vi "Navigation_Main_r1.2(new math for dist calc).vi"() -> ()   [LabVIEW 2015]
uses:
  <vilib>/myRIO/Common/Instrument Driver Framework/Utilities/typedefs/Generic FPGA Reference.ctl
  <vilib>/myRIO/Common/Instrument Driver Framework/Utilities/typedefs/myRIO v1.0 Reference.ctl
  <vilib>/myRIO/Common/Instrument Driver Framework/Utilities/typedefs/Hardware Version Enum.ctl
  <vilib>/myRIO/Common/Instrument Driver Framework/Utilities/typedefs/myRIO Generic Hardware Reference.ctl
  <vilib>/userdefined/High Color/nirio_resource_hc.ctl
  <vilib>/myRIO/Instrument Drivers/Onboard IO/PWM/typedefs/PWM Configuration.ctl
  <vilib>/myRIO/Instrument Drivers/Onboard IO/PWM/PWM.lvlib
  <vilib>/myRIO/Common/Instrument Driver Framework/myRIO v1.0/PWM/typedefs/PWM Channels Enum.ctl
  <vilib>/myRIO/Instrument Drivers/Onboard IO/PWM/typedefs/PWM Reference.ctl
  <vilib>/myRIO/Instrument Drivers/Onboard IO/PWM/vis/myRIO PWM Open.xnode
  <vilib>/myRIO/Common/Instrument Driver Framework/myRIO v1.0/PWM/vis/myRIO v1.1 Open PWM.vi
  <vilib>/rvi/interface/nirviOpenFPGA/nirviOpenFPGA.xnode
  <vilib>/myRIO/Instrument Drivers/Utilities/Utilities.lvlib
  <vilib>/rvi/interface/nirviReadWriteControl/nirviReadWriteControl.xnode
  NiFpgaLv.dll
  <vilib>/Utility/error.llb/Error Cluster From Error Code.vi
  <vilib>/rvi/interface/Simulation/niFpgaSimulationCallBeginRW.vi
  <vilib>/rvi/errors/niLvFpgaAdjustHostInterfaceError.vi
  Navi/E/FPGA Bitfiles/NavigationProjec_FPGATarget2_FPGAMainNavigati_PWPHW8gwDxI.lvbitx
  <vilib>/FPGAPlugInAG/myRIO-1900/niLvFpga_Open_myRIO-1900.vi
  <vilib>/rvi/interface/common/dynamic/niFpgaDynamicAddResources.vi
panel:
  out "max v":dbl
  out "v left wheel":dbl
  out "v right wheel":dbl
  out "Phi desired":dbl
  out "Omega":dbl format="%.2f"
  in  "Goal Position Y":dbl=5.0
  out "x position":dbl
  out "y position":dbl
  out "Scale":dbl=1.0
  out "Reset X Y":dbl
  out "Desired Velocity":dbl
  out "track width(ft)":dbl=4.0
  out "phi current":dbl
  out "robot desired velocity x component\n u1 (ft/s)":dbl
  out "robot desired velocity y component\n u2 (ft/s)":dbl
  out "RM Distance (ft)":dbl
  out "RR Distance (ft)":dbl
  out "LF Distance (ft)":dbl
  out "LM Distance (ft)":dbl
  out "RF Distance (ft)":dbl
  out "LR Distance (ft)":dbl
  out "Tick Count(mSec) 2":u32 caption="Tick Count(mSec)"
  out "Right Setpoint":dbl
  out "Left Setpoint":dbl
  in  "Start Position Y":dbl=5.0
  in  "Goal Position X":dbl=5.0
  in  "Start Position X":dbl=1.0
  in  "All Stop":bool
  in  "Left Side PID Gains":T1={"proportional gain (Kc)"=0.002, "integral time (Ti, min)"=7e-07, "derivative time (Td, min)"=0.0} {"derivative time (Td, min)" format="%.8f"; "integral time (Ti, min)" format="%.8f"; "proportional gain (Kc)" format="%.8f"}
  in  "Left Side Output Range":cluster{"output high":dbl, "output low":dbl}={"output high"=0.13333, "output low"=-0.13333} {"output low" format="%.5f"; "output high" format="%.5f"}
  in  "Right Side PID Gains":T1={"proportional gain (Kc)"=0.002, "integral time (Ti, min)"=7e-07, "derivative time (Td, min)"=0.0} {"derivative time (Td, min)" format="%.8f"; "integral time (Ti, min)" format="%.8f"; "proportional gain (Kc)" format="%.8f"}
  in  "Right Side Output Range":cluster{"output high":dbl, "output low":dbl}={"output high"=0.13333, "output low"=-0.13333} {"output low" format="%.5f"; "output high" format="%.5f"}
  out "Left PWM":dbl
  out "Right PWM":dbl
  out "LF Rot Velocity (rot/s)":dbl
  out "LM Rot Velocity (rot/s)":dbl
  out "LR Rot Velocity (rot/s)":dbl
  out "RR Rot Velocity (rot/s)":dbl
  out "RM Linear Velocity (rot/s)":dbl
  out "RF Linear Velocity (rot/s)":dbl
  in  "Encoder Reset":bool
  out "SYS.SELECTA":u8 format="%08b"
  out "ENC.B_c.CNTR":i32
  out "ENC.B_b.CNTR":i32
  out "ENC.B_a.CNTR":i32
  out "ENC.A_c.CNTR":i32
  out "ENC.A_b.CNTR":i32
  out "ENC.A_a.CNTR":i32
  out "Current Rot Velocity (rot/s)":T2(graph)
  # "Motor Control Parameters"
  # "Press Go when Start and Goal Are Set"
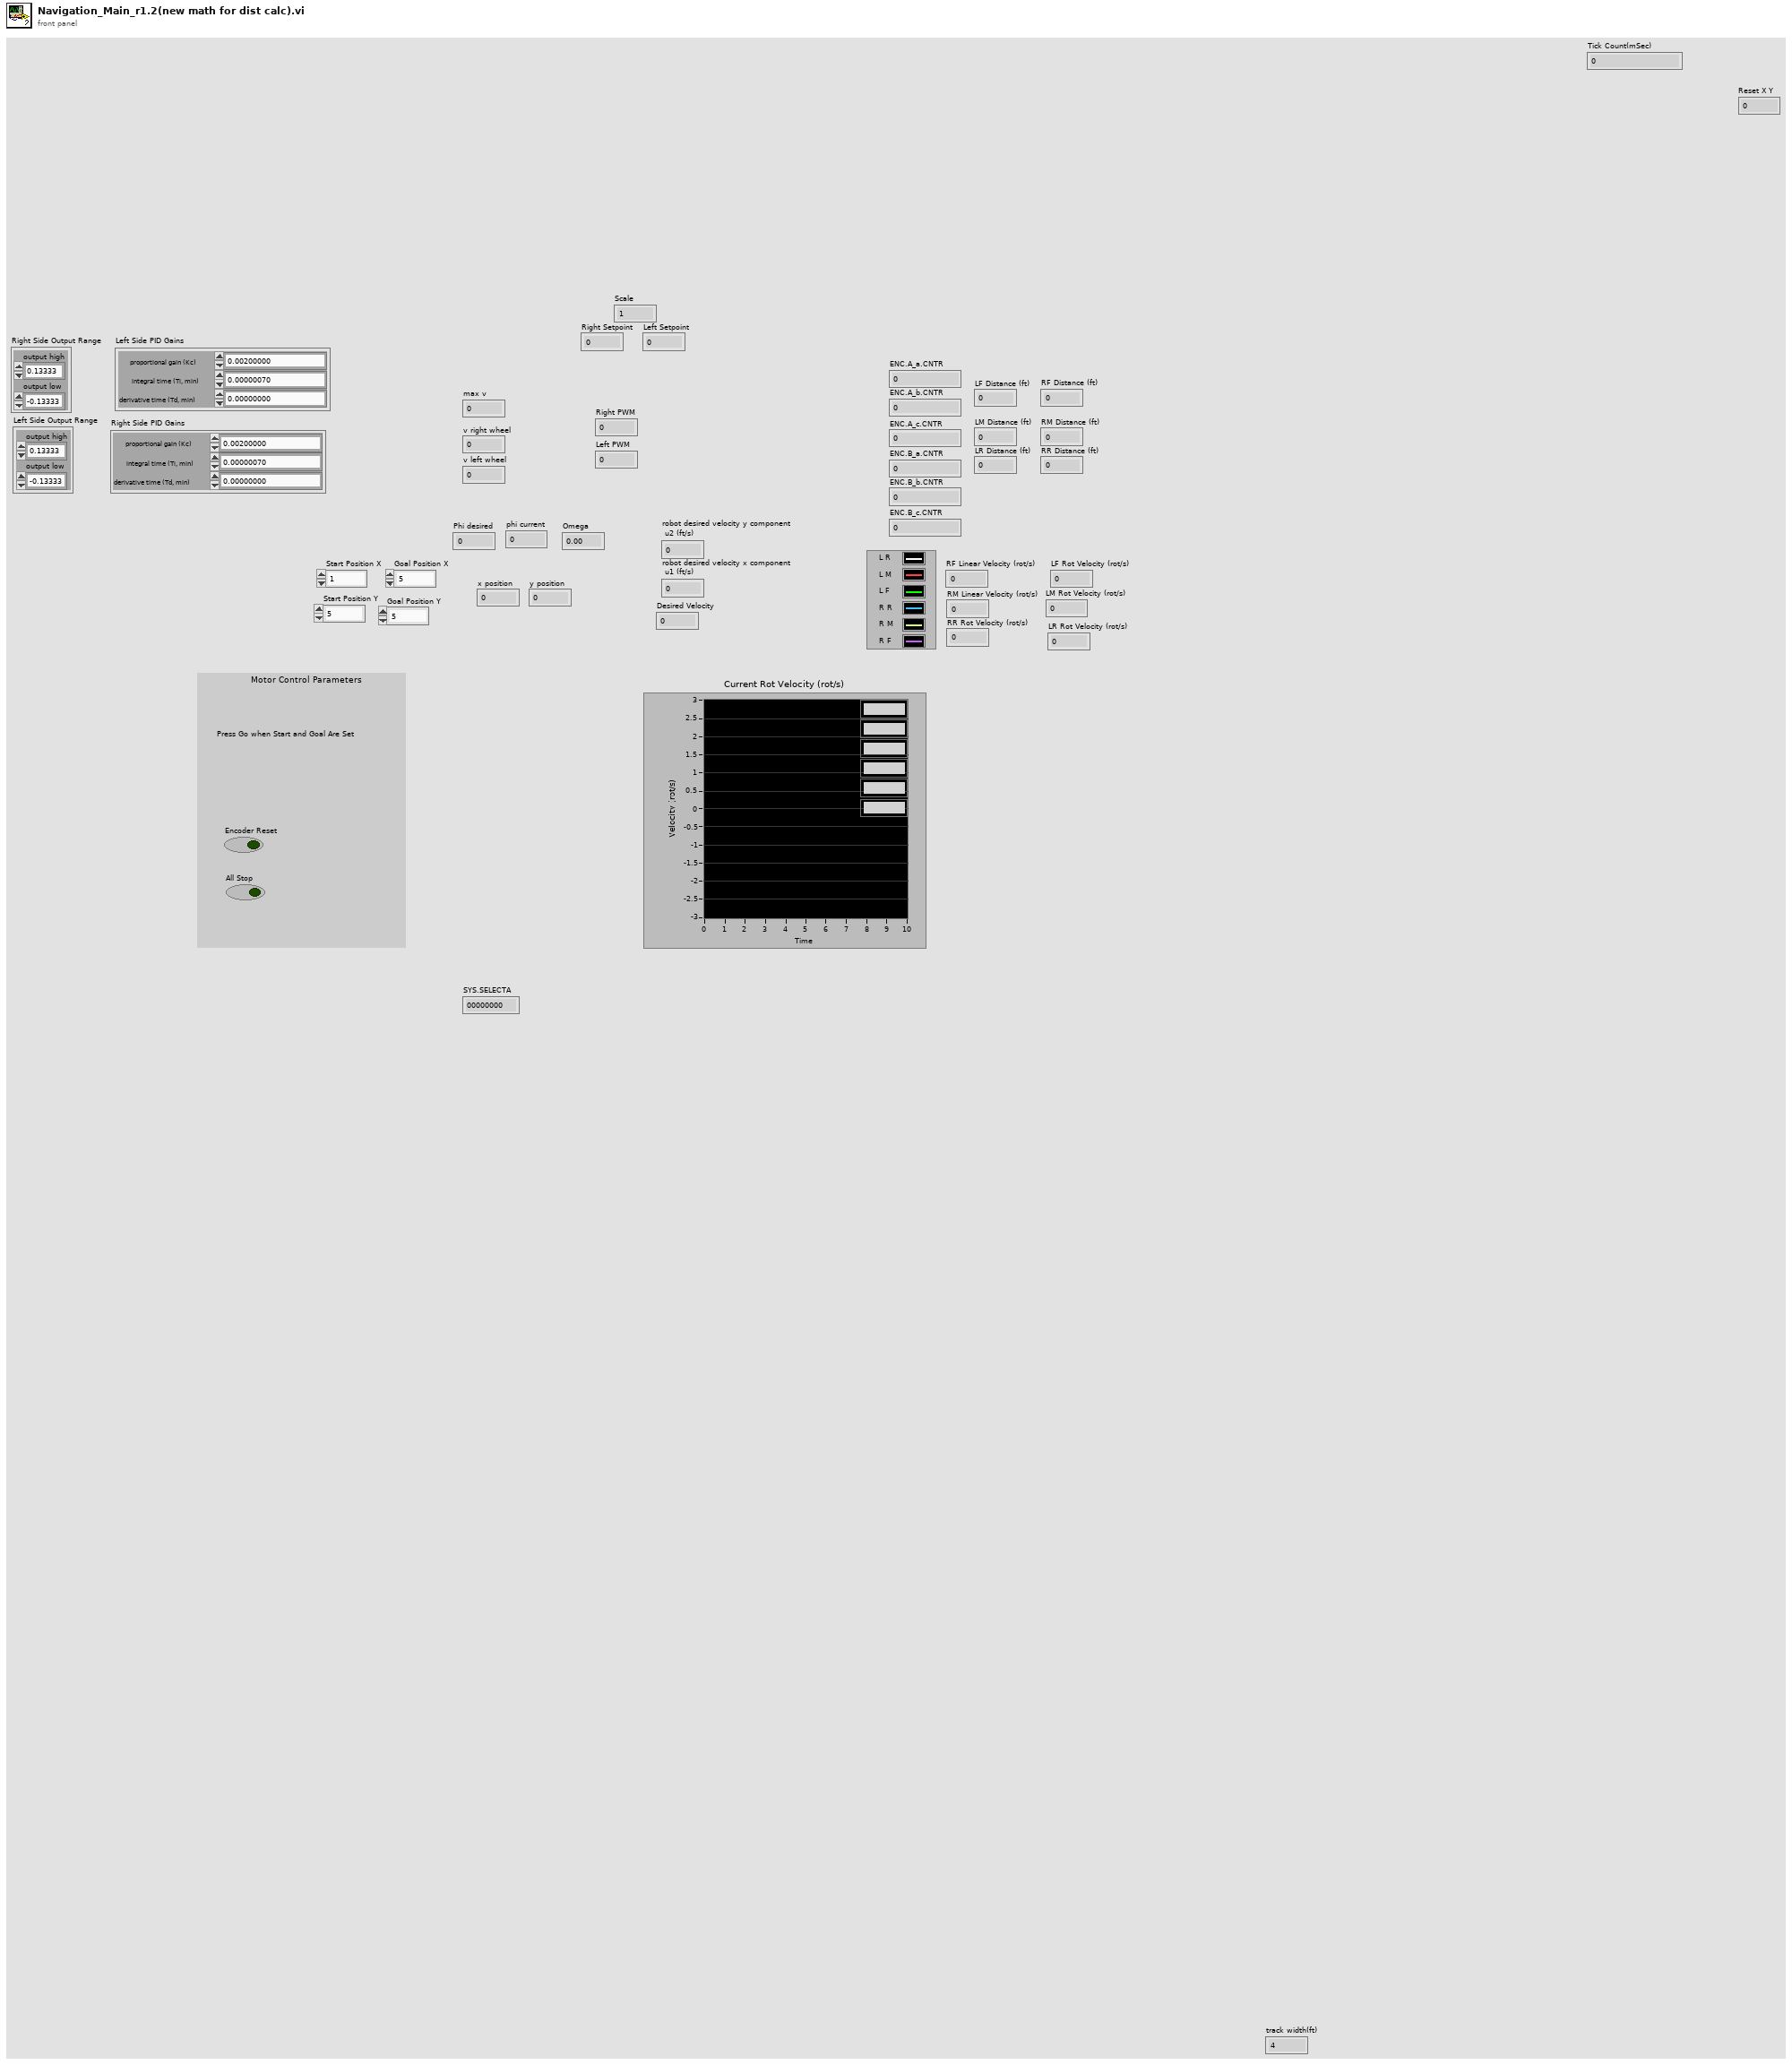
[diagram p1: front panel]
types:
  T1 = cluster{"proportional gain (Kc)":dbl, "integral time (Ti, min)":dbl, "derivative time (Td, min)":dbl}
  T2 = cluster{"Rotational Velocity (RPS)":dbl, "Rotational Velocity (RPS)":dbl, "Rotational Velocity (RPS)":dbl, "Rotational Velocity (RPS)":dbl, "Rotational Velocity (RPS)":dbl, "Rotational Velocity (RPS)":dbl}
  T3 = typedef "nirio_resource_hc.ctl" = tag
  T4 = typedef "Hardware Version Enum.ctl" = enum16{"Unknown", "myRIO-1900", "myRIO-1950", "roboRIO"}
  T5 = typedef "PWM.lvlib/PWM Reference.ctl" = cluster{"myRIO Reference":T6, "PWM Channels Enum":T9, "PWM Configuration":T10}
  T6 = typedef "myRIO Generic Hardware Reference.ctl" = cluster{"myRIO Model":T4, "myRIO Hardware Reference":T7}
  T7 = typedef "myRIO v1.0 Reference.ctl" = cluster{"Generic FPGA Reference":T8, "Allow multiple opens":bool}
  T8 = typedef "Generic FPGA Reference.ctl" = refnum<k20>
  T9 = typedef "PWM Channels Enum.ctl" = enum16{"Not Connected", "C/PWM0", "C/PWM1", "A/PWM0", "A/PWM1", "A/PWM2", "B/PWM0", "B/PWM1", "B/PWM2", "PWM/PWM0", "PWM/PWM1", "PWM/PWM2", "PWM/PWM3", "PWM/PWM4", "PWM/PWM5", "PWM/PWM6", "PWM/PWM7", "PWM/PWM8", "PWM/PWM9"}
  T10 = typedef "PWM.lvlib/PWM Configuration.ctl" = cluster{"Frequency":dbl, "Duty Cycle":dbl}
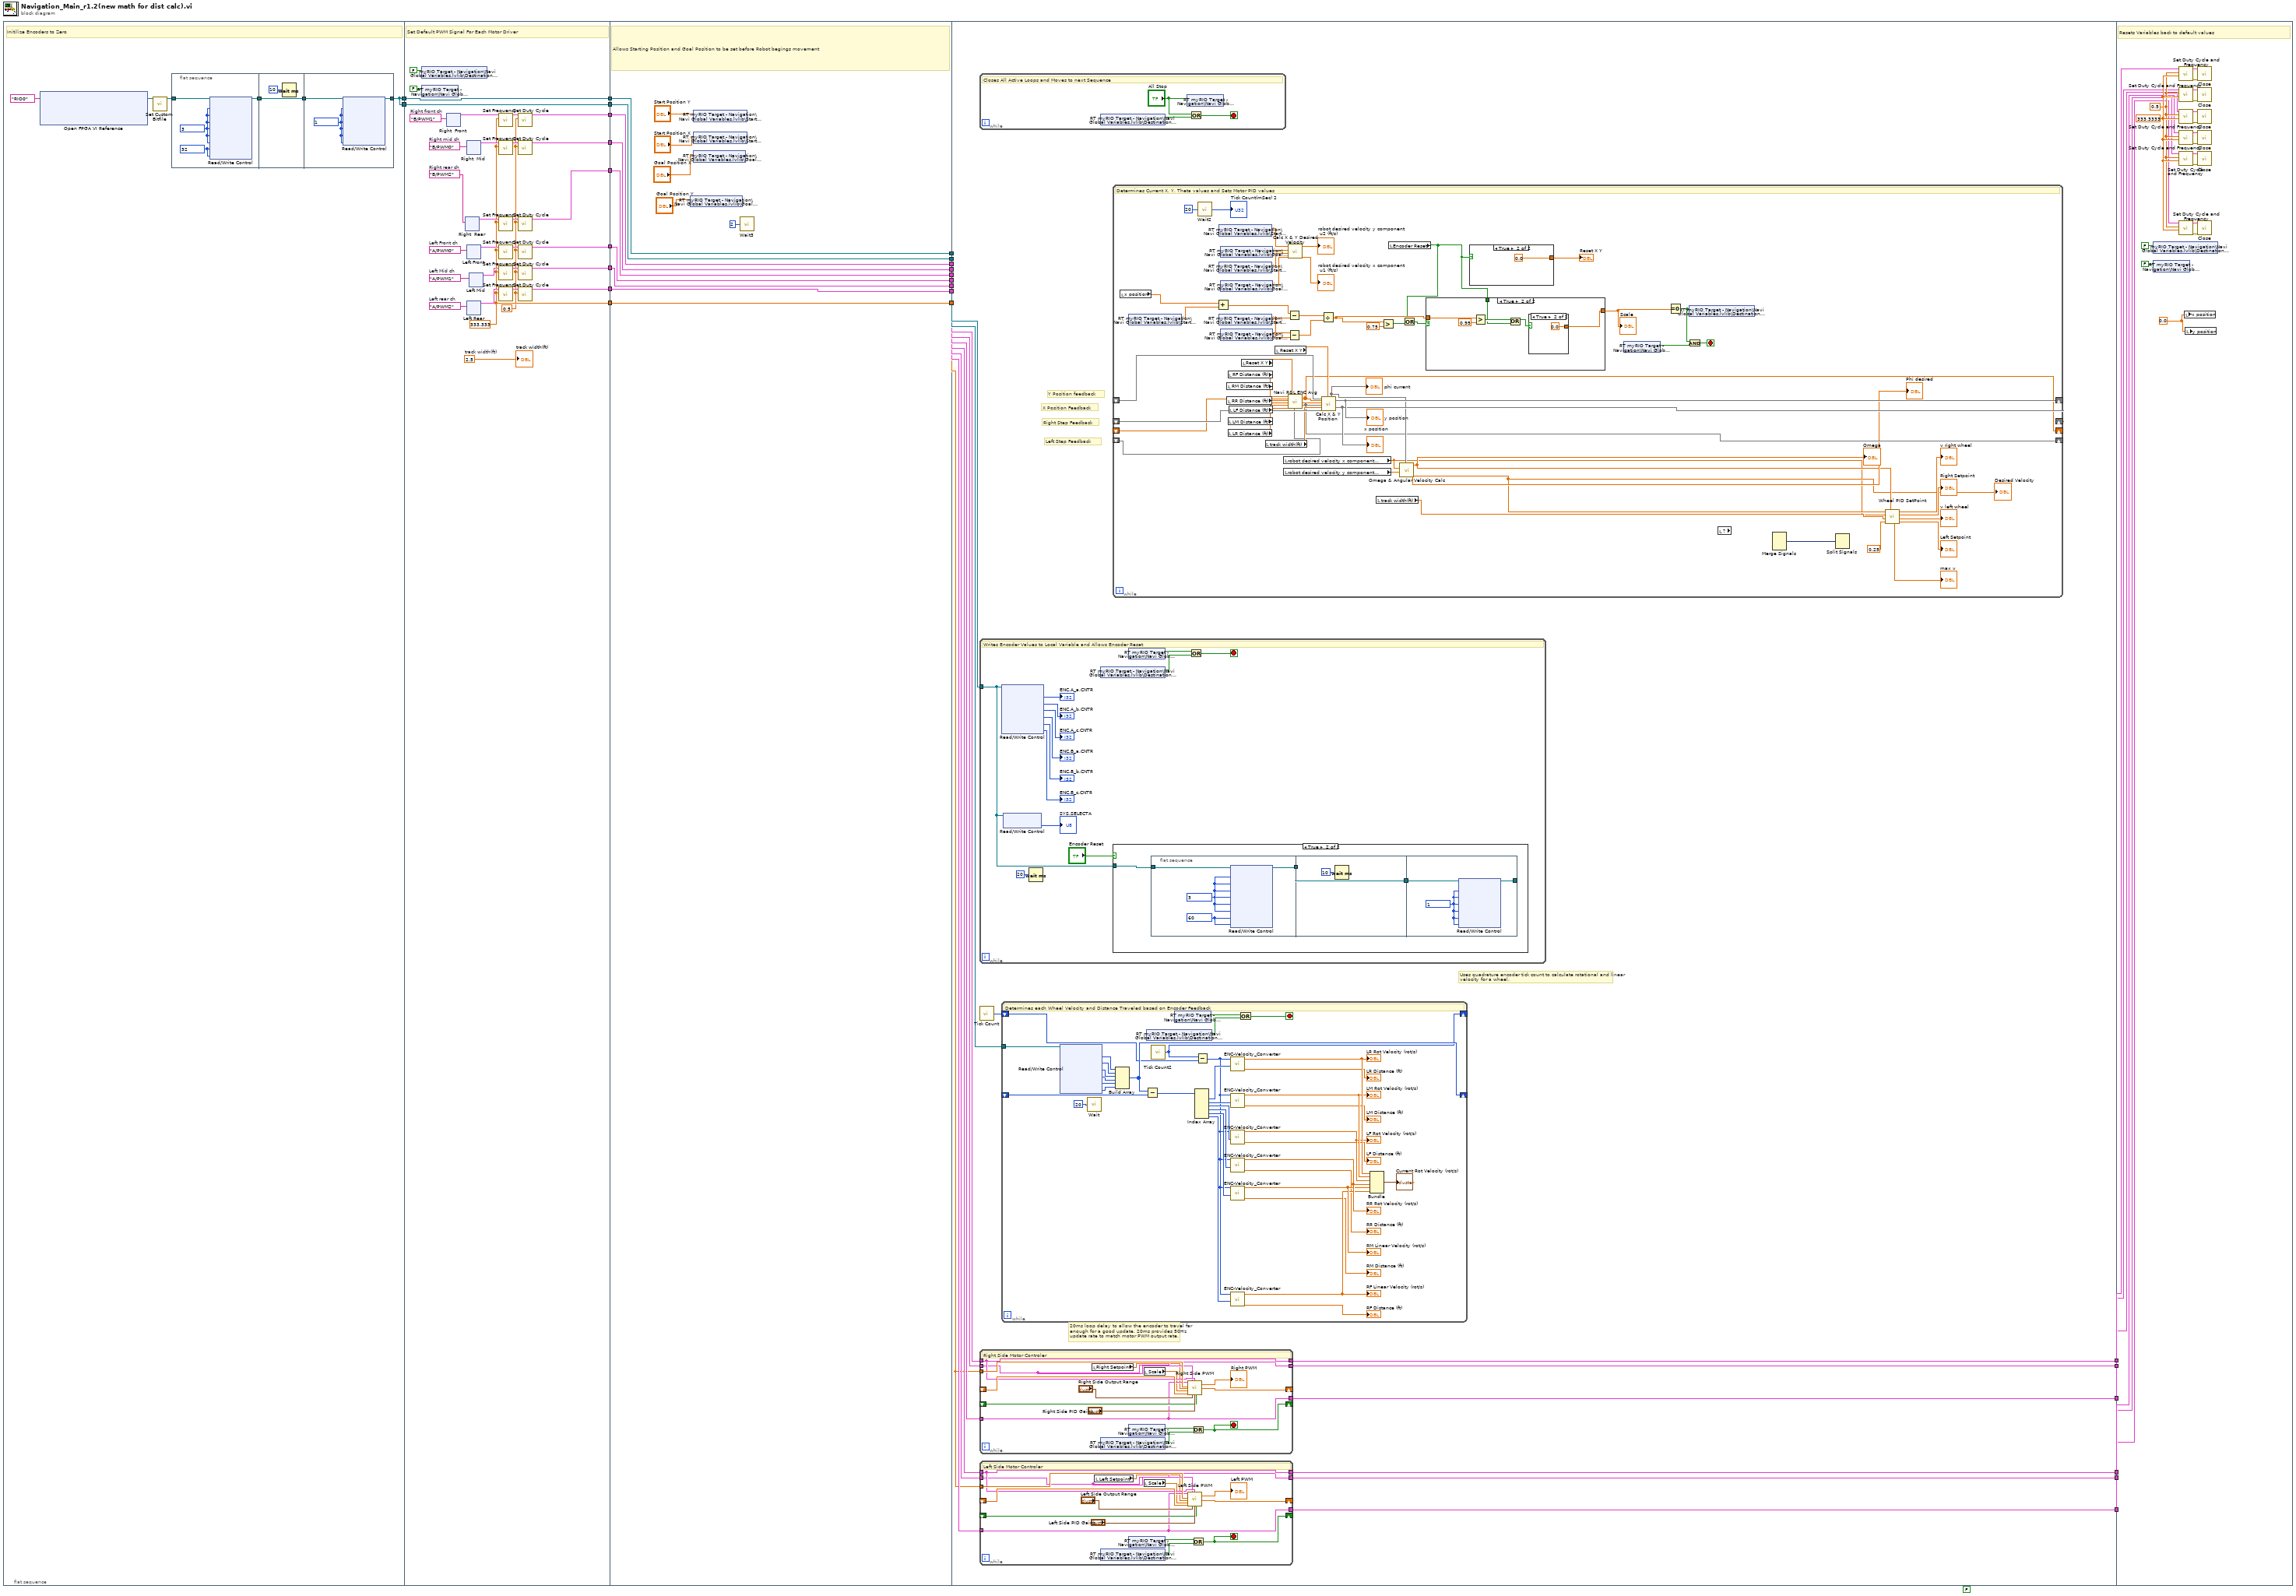
[diagram p0: block diagram]
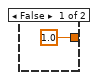
[diagram p2: hidden frame]
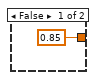
[diagram p3: hidden frame]
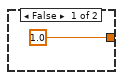
[diagram p4: hidden frame]
diagram:
  (unwired) FALSE ("stop")
  n1 = flat-sequence {
    tunnel: [w29] -> w26
    tunnel: [w29] -> w25
    tunnel: [w60] -> w24
    tunnel: [w55] -> w23
    tunnel: [w51] -> w22
    tunnel: [w50] -> w21
    tunnel: [w49] -> w20
    tunnel: [w48] -> w19
    tunnel: [w47] -> w18
    tunnel: [w46] -> w17
    tunnel: w26 -> [w45]
    tunnel: [w45] -> w16
    tunnel: w25 -> [w46]
    tunnel: w24 -> [w182]
    tunnel: [w182] -> w15
    tunnel: w23 -> [w181]
    tunnel: [w181] -> w14
    tunnel: w22 -> [w180]
    tunnel: [w180] -> w13
    tunnel: w21 -> [w179]
    tunnel: [w179] -> w12
    tunnel: w20 -> [w178]
    tunnel: [w178] -> w11
    tunnel: w19 -> [w177]
    tunnel: [w177] -> w10
    tunnel: w18 -> [w176]
    tunnel: [w176] -> w9
    tunnel: w17 -> [w175]
    tunnel: [w175] -> w8
    tunnel: w16 -> [w174]
    tunnel: [w174] -> w7
    tunnel: w15 -> [w189]
    tunnel: w14 -> [w190]
    tunnel: w13 -> [w195]
    tunnel: w12 -> [w194]
    tunnel: w11 -> [w193]
    tunnel: w10 -> [w192]
    tunnel: w9 -> [w191]
    tunnel: w8 -> [w197]
    tunnel: w7 -> [w196]
    tunnel: [w188] -> w6
    tunnel: [w187] -> w5
    tunnel: [w186] -> w4
    tunnel: [w185] -> w3
    tunnel: [w184] -> w2
    tunnel: [w183] -> w1
    tunnel: w6 -> [w369]
    tunnel: w5 -> [w368]
    tunnel: w4 -> [w367]
    tunnel: w3 -> [w366]
    tunnel: w2 -> [w365]
    tunnel: w1 -> [w364]
    frame #0 {
      # "Initilize Encoders to Zero"
      n2 = xnode "Open FPGA VI Reference"("resource name"=tag "RIO0") -> ("FPGA VI Reference Out"=w28:refnum<k20>)  [unwired: 1 in, 1 out]
      n3 = call <vilib>:"Set Custom Bitfile.vi"("Custom FPGA Reference In"=w28) -> ("Custom FPGA Reference Out"=w30:refnum<k20>)  [unwired: 9 in, 1 out]
      n4 = flat-sequence {
        tunnel: w30 -> [w35]
        tunnel: [w33] -> w32
        tunnel: w32 -> [w37]
        tunnel: [w37] -> w31
        tunnel: w31 -> [w40]
        tunnel: [w39] -> w29
        frame #0 {
          w34 = u8 32 ("SYS.SELECTA")
          w36 = u8 3 ("ENC.B_c.CNFG")
          n5 = xnode "Read/Write Control"("FPGA VI Reference In"=w35, "ENC.A_a.CNFG"=w36, "ENC.A_b.CNFG"=w36, "ENC.A_c.CNFG"=w36, "ENC.B_a.CNFG"=w36, "ENC.B_b.CNFG"=w36, "ENC.B_c.CNFG"=w36, "SYS.SELECTA"=w34, "SYS.SELECTB"=w34) -> ("FPGA VI Reference Out"=w33:refnum<k20>)  [unwired: 1 in, 1 out]
        }
        frame #1 {
          n6 = Wait (ms)(milliseconds to wait=u32 10) -> ()  [unwired: 1 out]
        }
        frame #2 {
          w41 = u8 1 ("ENC.B_c.CNFG")
          n7 = xnode "Read/Write Control"("FPGA VI Reference In"=w40, "ENC.A_a.CNFG"=w41, "ENC.A_b.CNFG"=w41, "ENC.A_c.CNFG"=w41, "ENC.B_a.CNFG"=w41, "ENC.B_b.CNFG"=w41, "ENC.B_c.CNFG"=w41) -> ("FPGA VI Reference Out"=w39:refnum<k20>)  [unwired: 1 in, 1 out]
        }
      }
    }
    frame #1 {
      w42 = 2.5  # track width(ft)
      w52 = 0.5 ("Duty Cycle")
      w60 = 333.333 ("Frequency [Hz]")
      w67 = tag "B/PWM2"  # Right rear ch
      w68 = tag "B/PWM0"  # Right mid ch
      w69 = tag "B/PWM1"  # Right front ch
      w70 = tag "A/PWM2"  # Left rear ch
      w71 = tag "A/PWM0"  # Left Front ch
      w72 = tag "A/PWM1"  # Left Mid ch
      # "Set Default PWM Signal For Each Motor Driver"
      n8 = shared-variable "RT myRIO Target - Navigation\\Navi Global Variables.lvlib\\Destination Reached"(FALSE) -> ()  [unwired: 1 in, 1 out]
      n9 = shared-variable "RT myRIO Target - Navigation\\Navi Global Variables.lvlib\\All Stop"(FALSE) -> ()  [unwired: 1 in, 1 out]
      n10 = xnode "Right  Front"("Channel Name"=w69) -> ("PWM Ref Out"=w63:T5)  [unwired: 2 in, 1 out]
      n11 = xnode "Right  Rear"("Channel Name"=w67) -> ("PWM Ref Out"=w61:T5)  [unwired: 2 in, 1 out]
      n12 = xnode "Right  Mid"("Channel Name"=w68) -> ("PWM Ref Out"=w62:T5)  [unwired: 2 in, 1 out]
      n13 = xnode "Left Front"("Channel Name"=w71) -> ("PWM Ref Out"=w65:T5)  [unwired: 2 in, 1 out]
      n14 = xnode "Left Rear"("Channel Name"=w70) -> ("PWM Ref Out"=w64:T5)  [unwired: 2 in, 1 out]
      n15 = xnode "Left Mid"("Channel Name"=w72) -> ("PWM Ref Out"=w66:T5)  [unwired: 2 in, 1 out]
      n16 = call <vilib>:"Set Frequency.vi"("Frequency [Hz]"=w60, "PWM Ref In"=w63) -> ("PWM Ref Out"=w56:T5)  [unwired: 7 in, 1 out]
      n17 = call <vilib>:"Set Frequency.vi"("Frequency [Hz]"=w60, "PWM Ref In"=w62) -> ("PWM Ref Out"=w57:T5)  [unwired: 7 in, 1 out]
      n18 = call <vilib>:"Set Frequency.vi"("Frequency [Hz]"=w60, "PWM Ref In"=w61) -> ("PWM Ref Out"=w58:T5)  [unwired: 7 in, 1 out]
      n19 = call <vilib>:"Set Frequency.vi"("Frequency [Hz]"=w60, "PWM Ref In"=w65) -> ("PWM Ref Out"=w53:T5)  [unwired: 7 in, 1 out]
      n20 = call <vilib>:"Set Frequency.vi"("Frequency [Hz]"=w60, "PWM Ref In"=w66) -> ("PWM Ref Out"=w59:T5)  [unwired: 7 in, 1 out]
      n21 = call <vilib>:"Set Frequency.vi"("Frequency [Hz]"=w60, "PWM Ref In"=w64) -> ("PWM Ref Out"=w54:T5)  [unwired: 7 in, 1 out]
      n22 = call <vilib>:"Set Duty Cycle.vi"("Duty Cycle"=w52, "PWM Ref In"=w56) -> ("PWM Ref Out"=w51:T5)  [unwired: 7 in, 1 out]
      n23 = call <vilib>:"Set Duty Cycle.vi"("Duty Cycle"=w52, "PWM Ref In"=w57) -> ("PWM Ref Out"=w50:T5)  [unwired: 7 in, 1 out]
      n24 = call <vilib>:"Set Duty Cycle.vi"("Duty Cycle"=w52, "PWM Ref In"=w58) -> ("PWM Ref Out"=w49:T5)  [unwired: 7 in, 1 out]
      n25 = call <vilib>:"Set Duty Cycle.vi"("Duty Cycle"=w52, "PWM Ref In"=w53) -> ("PWM Ref Out"=w48:T5)  [unwired: 7 in, 1 out]
      n26 = call <vilib>:"Set Duty Cycle.vi"("Duty Cycle"=w52, "PWM Ref In"=w59) -> ("PWM Ref Out"=w47:T5)  [unwired: 7 in, 1 out]
      n27 = call <vilib>:"Set Duty Cycle.vi"("Duty Cycle"=w52, "PWM Ref In"=w54) -> ("PWM Ref Out"=w55:T5)  [unwired: 7 in, 1 out]
      "track width(ft)" <- w42
    }
    frame #2 {
      # "Allows Starting Position and Goal Position to be set before Robot begings movement"
      n28 = shared-variable "RT myRIO Target - Navigation\\Navi Global Variables.lvlib\\Goal Position Y"("Goal Position Y") -> ()  [unwired: 1 in, 1 out]
      n29 = shared-variable "RT myRIO Target - Navigation\\Navi Global Variables.lvlib\\Start Position Y"("Start Position Y") -> ()  [unwired: 1 in, 1 out]
      n30 = shared-variable "RT myRIO Target - Navigation\\Navi Global Variables.lvlib\\Start Position X"("Start Position X") -> ()  [unwired: 1 in, 1 out]
      n31 = shared-variable "RT myRIO Target - Navigation\\Navi Global Variables.lvlib\\Goal Position X"("Goal Position X") -> ()  [unwired: 1 in, 1 out]
      n32 = call "Wait3"("Count(mSec)"=u32 2) -> ()  [unwired: 1 out]
    }
    frame #3 {
      # "Left Step Feedback"
      # "Y Position feedback"
      # "Right Step Feedback"
      # "X Position Feedback"
      # "Uses quadrature encoder tick count to calculate rotational and linear velocity for a wheel."
      # "20ms loop delay to allow the encoder to travel far enough for a good update. 20ms provides 50Hz update rate to match motor PWM output rate."
      n33 = while {
        stop <- w269 stop-if-true
        # "Closes All Active Loops and Moves to next Sequence"
        n34 = shared-variable "RT myRIO Target - Navigation\\Navi Global Variables.lvlib\\Destination Reached"() -> (w267:bool)  [unwired: 1 in, 1 out]
        n35 = shared-variable "RT myRIO Target - Navigation\\Navi Global Variables.lvlib\\All Stop"("All Stop") -> ()  [unwired: 1 in, 1 out]
        n36 = Or(x="All Stop", y=w267) -> (x .or. y?=w269:bool)
      }
      n37 = while {
        tunnel: w197 -> [w303]
        stop <- w300 stop-if-true
        # "Writes Encoder Values to Local Variable and Allows Encoder Reset"
        n38 = xnode "Read/Write Control"("FPGA VI Reference In"=w303) -> ("ENC.A_a.CNTR"=→"ENC.A_a.CNTR":u32, "ENC.A_b.CNTR"=→"ENC.A_b.CNTR":u32, "ENC.A_c.CNTR"=→"ENC.A_c.CNTR":u32, "ENC.B_a.CNTR"=→"ENC.B_a.CNTR":u32, "ENC.B_b.CNTR"=→"ENC.B_b.CNTR":u32, "ENC.B_c.CNTR"=→"ENC.B_c.CNTR":u32)  [unwired: 1 in, 2 out]
        n39 = xnode "Read/Write Control"("FPGA VI Reference In"=w303) -> ("SYS.SELECTA"=→"SYS.SELECTA":u8)  [unwired: 1 in, 2 out]
        n40 = Wait (ms)(milliseconds to wait=u32 20) -> ()  [unwired: 1 out]
        n41 = shared-variable "RT myRIO Target - Navigation\\Navi Global Variables.lvlib\\Destination Reached"() -> (w302:bool)  [unwired: 1 in, 1 out]
        n42 = case shown="True" "Encoder Reset" {
          tunnel: w303 -> [_ w313]
          frame False {
          }
          frame True {
            n43 = flat-sequence {
              tunnel: w313 -> [w318]
              tunnel: [w316] -> w315
              tunnel: w315 -> [w320]
              tunnel: [w320] -> w314
              tunnel: w314 -> [w323]
              tunnel: [w322] -> _
              frame #0 {
                w317 = u8 60 ("SYS.SELECTA")
                w319 = u8 3 ("ENC.B_c.CNFG")
                n44 = xnode "Read/Write Control"("FPGA VI Reference In"=w318, "ENC.A_a.CNFG"=w319, "ENC.A_b.CNFG"=w319, "ENC.A_c.CNFG"=w319, "ENC.B_a.CNFG"=w319, "ENC.B_b.CNFG"=w319, "ENC.B_c.CNFG"=w319, "SYS.SELECTA"=w317, "SYS.SELECTB"=w317) -> ("FPGA VI Reference Out"=w316:refnum<k20>)  [unwired: 1 in, 1 out]
              }
              frame #1 {
                n45 = Wait (ms)(milliseconds to wait=u32 10) -> ()  [unwired: 1 out]
              }
              frame #2 {
                w324 = u8 1 ("ENC.B_c.CNFG")
                n46 = xnode "Read/Write Control"("FPGA VI Reference In"=w323, "ENC.A_a.CNFG"=w324, "ENC.A_b.CNFG"=w324, "ENC.A_c.CNFG"=w324, "ENC.B_a.CNFG"=w324, "ENC.B_b.CNFG"=w324, "ENC.B_c.CNFG"=w324) -> ("FPGA VI Reference Out"=w322:refnum<k20>)  [unwired: 1 in, 1 out]
              }
            }
          }
        }
        n47 = shared-variable "RT myRIO Target - Navigation\\Navi Global Variables.lvlib\\All Stop"() -> (w301:bool)  [unwired: 1 in, 1 out]
        n48 = Or(x=w301, y=w302) -> (x .or. y?=w300:bool)
      }
      n49 = call "Tick Count"() -> ("Tick Count(uSec)"=w198:u32)
      n50 = while {
        tunnel: w195 -> [w292]
        tunnel: w194 -> [w291]
        tunnel: w193 -> [w290]
        tunnel: w189 -> [w299]
        shift-right: [w295] -> _
        shift-left: _ -> [w294]
        shift-right: [w287] -> _
        shift-left: _ -> [w293]
        tunnel: [w292] -> w188
        tunnel: [w291] -> w187
        tunnel: [w290] -> w186
        stop <- w287 stop-if-true
        # "Right Side Motor Controler"
        n51 = local read "Right Setpoint"() -> (w286:dbl)
        n52 = shared-variable "RT myRIO Target - Navigation\\Navi Global Variables.lvlib\\Destination Reached"() -> (w289:bool)  [unwired: 1 in, 1 out]
        n53 = shared-variable "RT myRIO Target - Navigation\\Navi Global Variables.lvlib\\All Stop"() -> (w288:bool)  [unwired: 1 in, 1 out]
        n54 = local read "Scale"() -> (w285:dbl)
        n55 = call "Right Side PWM.vi"("Right rear"=w290, "Frequency"=w299, "Right Side Setpoint"=w286, "Right Side Scale"=w285, "Right PID Feedback"=w294, "Right Mid"=w291, "Right Side Output Range"="Right Side Output Range", "Right Front"=w292, "Right Side PID Gains"="Right Side PID Gains", "Reset Right E.T."=w293) -> ("Right PWM"=→"Right PWM":dbl, "Right PID Output"=w295:dbl)  [unwired: 8 in]
        n56 = Or(x=w288, y=w289) -> (x .or. y?=w287:bool)
      }
      n57 = while {
        tunnel: w192 -> [w277]
        tunnel: w191 -> [w276]
        tunnel: w190 -> [w275]
        tunnel: w189 -> [w284]
        shift-right: [w280] -> _
        shift-left: _ -> [w279]
        shift-right: [w272] -> _
        shift-left: _ -> [w278]
        tunnel: [w277] -> w185
        tunnel: [w276] -> w184
        tunnel: [w275] -> w183
        stop <- w272 stop-if-true
        # "Left Side Motor Controler"
        n58 = local read "Left Setpoint"() -> (w271:dbl)
        n59 = shared-variable "RT myRIO Target - Navigation\\Navi Global Variables.lvlib\\Destination Reached"() -> (w274:bool)  [unwired: 1 in, 1 out]
        n60 = shared-variable "RT myRIO Target - Navigation\\Navi Global Variables.lvlib\\All Stop"() -> (w273:bool)  [unwired: 1 in, 1 out]
        n61 = local read "Scale"() -> (w270:dbl)
        n62 = call "Left Side PWM.vi"("Left rear"=w275, "Frequency"=w284, "Left Side Setpoint"=w271, "Left Side Scale"=w270, "Left PID Feedback"=w279, "Left Mid"=w276, "Left Side Output Range"="Left Side Output Range", "Left Front"=w277, "Left Side PID Gains"="Left Side PID Gains", "Reset Left E.T."=w278) -> ("Left PWM"=→"Left PWM":dbl, "Left PID Output"=w280:dbl)  [unwired: 8 in]
        n63 = Or(x=w273, y=w274) -> (x .or. y?=w272:bool)
      }
      n64 = while {
        shift-right: [w352] -> _
        shift-left: _ -> [w351]
        shift-right: [w349] -> _
        shift-left: w198 -> [w348]
        tunnel: w196 -> [w359]
        stop <- w344 stop-if-true
        # "Determines each Wheel Velocity and Distance Traveled based on Encoder Feedback"
        n65 = xnode "Read/Write Control"("FPGA VI Reference In"=w359) -> ("ENC.A_a.CNTR"=w358:u32, "ENC.A_b.CNTR"=w357:u32, "ENC.A_c.CNTR"=w356:u32, "ENC.B_a.CNTR"=w355:u32, "ENC.B_b.CNTR"=w354:u32, "ENC.B_c.CNTR"=w353:u32)  [unwired: 1 in, 2 out]
        n66 = call "Wait"("Count(mSec)"=u32 20) -> ()  [unwired: 1 out]
        n67 = Build Array(w358, w357, w356, w355, w354, w353) -> (w352:u32[])
        n68 = Subtract(x=w352, y=w351) -> (x-y=w350:u32[])
        n69 = shared-variable "RT myRIO Target - Navigation\\Navi Global Variables.lvlib\\Destination Reached"() -> (w346:bool)  [unwired: 1 in, 1 out]
        n70 = call "Tick Count2"() -> ("Tick Count(uSec)"=w349:u32)
        n71 = shared-variable "RT myRIO Target - Navigation\\Navi Global Variables.lvlib\\All Stop"() -> (w345:bool)  [unwired: 1 in, 1 out]
        n72 = Index Array(array=w350) -> (element #1=w343:u32, element #2=w340:u32, element #3=w338:u32, element #4=w336:u32, element #5=w334:u32, element #6=w331:u32)  [unwired: 6 in]
        n73 = Subtract(x=w349, y=w348) -> (x-y=w332:u32)
        n74 = call "ENC-Velocity_Converter.vi"("delta  Encoder Count"=w343, "dt (uSec)"=w332) -> ("Distance (ft)"=→"LR Distance (ft)":dbl, "Rotational Velocity (RPS)"=w342:dbl)  [unwired: 7 in, 1 out]
        "LR Rot Velocity (rot/s)" <- w342
        n75 = call "ENC-Velocity_Converter.vi"("delta  Encoder Count"=w340, "dt (uSec)"=w332) -> ("Distance (ft)"=→"LM Distance (ft)":dbl, "Rotational Velocity (RPS)"=w341:dbl)  [unwired: 7 in, 1 out]
        "LM Rot Velocity (rot/s)" <- w341
        n76 = call "ENC-Velocity_Converter.vi"("delta  Encoder Count"=w338, "dt (uSec)"=w332) -> ("Distance (ft)"=→"LF Distance (ft)":dbl, "Rotational Velocity (RPS)"=w339:dbl)  [unwired: 7 in, 1 out]
        "LF Rot Velocity (rot/s)" <- w339
        n77 = call "ENC-Velocity_Converter.vi"("delta  Encoder Count"=w336, "dt (uSec)"=w332) -> ("Distance (ft)"=→"RR Distance (ft)":dbl, "Rotational Velocity (RPS)"=w337:dbl)  [unwired: 7 in, 1 out]
        "RR Rot Velocity (rot/s)" <- w337
        n78 = call "ENC-Velocity_Converter.vi"("delta  Encoder Count"=w334, "dt (uSec)"=w332) -> ("Distance (ft)"=→"RM Distance (ft)":dbl, "Rotational Velocity (RPS)"=w335:dbl)  [unwired: 7 in, 1 out]
        "RM Linear Velocity (rot/s)" <- w335
        n79 = call "ENC-Velocity_Converter.vi"("delta  Encoder Count"=w331, "dt (uSec)"=w332) -> ("Distance (ft)"=→"RF Distance (ft)":dbl, "Rotational Velocity (RPS)"=w333:dbl)  [unwired: 7 in, 1 out]
        "RF Linear Velocity (rot/s)" <- w333
        n80 = Or(x=w345, y=w346) -> (x .or. y?=w344:bool)
        n81 = Bundle("Rotational Velocity (RPS)"=w342, "Rotational Velocity (RPS)"=w341, "Rotational Velocity (RPS)"=w339, "Rotational Velocity (RPS)"=w337, "Rotational Velocity (RPS)"=w335, "Rotational Velocity (RPS)"=w333) -> (→"Current Rot Velocity (rot/s)":T2)  [unwired: 1 in]
      }
      n82 = while {
        shift-right: [w241] -> _
        shift-left: _ -> [w243]
        shift-right: [w217] -> _
        shift-left: _ -> [w239]
        shift-right: [w242] -> _
        shift-left: _ -> [w244]
        shift-right: [w216] -> _
        shift-left: _ -> [w238]
        stop <- w251 stop-if-true
        # "Determines Current X, Y, Theta values and Sets Motor PID values"
        n83 = local read "x position"() -> (w206:dbl)
        n84 = shared-variable "RT myRIO Target - Navigation\\Navi Global Variables.lvlib\\Start Position X"() -> (w205:dbl)  [unwired: 1 in, 1 out]
        n85 = call "Wait2"("Count(mSec)"=u32 20) -> ("Tick Count(mSec)"=→"Tick Count(mSec) 2":u32)
        n86 = Add(x=w206, y=w205) -> (x+y=w204:dbl)
        n87 = shared-variable "RT myRIO Target - Navigation\\Navi Global Variables.lvlib\\Start Position Y"() -> (w250:dbl)  [unwired: 1 in, 1 out]
        n88 = shared-variable "RT myRIO Target - Navigation\\Navi Global Variables.lvlib\\Start Position X"() -> (w248:dbl)  [unwired: 1 in, 1 out]
        n89 = shared-variable "RT myRIO Target - Navigation\\Navi Global Variables.lvlib\\Start Position X"() -> (w218:dbl)  [unwired: 1 in, 1 out]
        n90 = shared-variable "RT myRIO Target - Navigation\\Navi Global Variables.lvlib\\Goal Position Y"() -> (w249:dbl)  [unwired: 1 in, 1 out]
        n91 = shared-variable "RT myRIO Target - Navigation\\Navi Global Variables.lvlib\\Goal Position X"() -> (w247:dbl)  [unwired: 1 in, 1 out]
        n92 = shared-variable "RT myRIO Target - Navigation\\Navi Global Variables.lvlib\\Goal Position X"() -> (w219:dbl)  [unwired: 1 in, 1 out]
        n93 = local read "RM Distance (ft)"() -> (w236:dbl)
        n94 = local read "RR Distance (ft)"() -> (w235:dbl)
        n95 = local read "RF Distance (ft)"() -> (w237:dbl)
        n96 = local read "LM Distance (ft)"() -> (w233:dbl)
        n97 = local read "LR Distance (ft)"() -> (w232:dbl)
        n98 = local read "LF Distance (ft)"() -> (w234:dbl)
        n99 = local read "Reset X Y"() -> (w221:dbl)
        n100 = local read "track width(ft)"() -> (w240:dbl)
        n101 = local read "Reset X Y"() -> (w220:dbl)
        n102 = local read "robot desired velocity x component\n u1 (ft/s)"() -> (w202:dbl)
        n103 = local read "robot desired velocity y component\n u2 (ft/s)"() -> (w230:dbl)
        n104 = Subtract(x=w204, y=w218) -> (x-y=w225:dbl)
        n105 = Subtract(x=w219, y=w218) -> (x-y=w222:dbl)
        n106 = call "Calc X & Y Desired Velocity.vi"("x goal"=w247, "x start"=w248, "Y Goal"=w249, "Y Position"=w250) -> ("robot desired velocity x component\n u1 (ft/s)"=→"robot desired velocity x component\n u1 (ft/s)":dbl, "robot desired velocity y component\n u2 (ft/s)"=→"robot desired velocity y component\n u2 (ft/s)":dbl)  [unwired: 6 in]
        n107 = Divide(x=w225, y=w222) -> (x/y=w224:dbl)
        n108 = local read "track width(ft)"() -> (w208:dbl)
        n109 = Greater?(x=w224, y=0.75) -> (0:w223:bool)
        n110 = local read "Encoder Reset"() -> (w200:bool)
        n111 = Or(x=w200, y=w223) -> (x .or. y?=w201:bool)
        n112 = case shown="True" w201 {
          tunnel: w224 -> [_ w262]
          tunnel: [1.0 w259] -> w214
          tunnel: w200 -> [_ w257]
          frame False {
          }
          frame True {
            n113 = Greater?(x=w262, y=0.95) -> (0:w260:bool)
            n114 = Or(x=w260, y=w257) -> (x .or. y?=w258:bool)
            n115 = case shown="True" w258 {
              tunnel: [0.85 0.0] -> w259
              frame False {
              }
              frame True {
              }
            }
          }
        }
        "Scale" <- w214
        n116 = case shown="True" w200 {
          tunnel: [1.0 0.0] -> w226
          frame False {
          }
          frame True {
          }
        }
        "Reset X Y" <- w226
        n117 = shared-variable "RT myRIO Target - Navigation\\Navi Global Variables.lvlib\\All Stop"() -> (w253:bool)  [unwired: 1 in, 1 out]
        n118 = Equal To 0?(x=w214) -> (x = 0?=w252:bool)
        n119 = And(x=w252, y=w253) -> (x .and. y?=w251:bool)
        n120 = shared-variable "RT myRIO Target - Navigation\\Navi Global Variables.lvlib\\Destination Reached"(w252) -> ()  [unwired: 1 in, 1 out]
        n121 = local read item#-1() -> ()  [unwired: 1 out]
        n122 = Merge Signals() -> (w199:dynamicdata)  [unwired: 5 in]
        n123 = Split Signals(w199) -> ()  [unwired: 4 in, 4 out]
        n124 = call "Navi R&L ENC Avg.vi"(0:w237, "encoder step sub vi input"=w236, 2:w235, 3:w234, 4:w233, 5:w232, 6:w221, "Reset X Y"=w239, 9:w238, 17:w231) -> ("encoder step sub vi output"=w217:dbl[], 18:w216)  [unwired: 8 in]
        n125 = call "Calc X & Y Position.vi"(0:w244, 1:w217, 3:w216, 4:w240, "x & y position input array"=w243, 8:w220) -> ("phi step"=w231:dbl, 12:w229, 15:w242, 18:w241)  [unwired: 9 in, 1 out]
        "phi current" <- w229
        "y position" <- w242
        "x position" <- w241
        n126 = call "Omega & Angular Velocity Calc.vi"("Phi Current"=w229, "Desired Y Velocity u2"=w230, "Desired X Velocity u1"=w202) -> ("Desired Velocity"=w203:dbl, "Phi desired"=→"Phi desired":dbl, "Omega"=w209:dbl)  [unwired: 6 in]
        "Desired Velocity" <- w203
        "Omega" <- w209
        n127 = call "Wheel PID SetPoint.vi"("Omega"=w209, "Wheel Radius"=0.25, "Track Width"=w208, "x sign"=w202, "Desired Velocity"=w203) -> ("Left Side Setpoint"=→"Left Setpoint":dbl, "v left wheel"=→"v left wheel":dbl, "Right Side Setpoint"=→"Right Setpoint":dbl, "v right wheel"=→"v right wheel":dbl, "max v"=→"max v":dbl)  [unwired: 2 in]
      }
    }
    frame #4 {
      w361 = 0.0
      w370 = 0.5
      w371 = 333.3333
      # "Resets Variables back to default values"
      n128 = shared-variable "RT myRIO Target - Navigation\\Navi Global Variables.lvlib\\Destination Reached"(FALSE) -> ()  [unwired: 1 in, 1 out]
      n129 = shared-variable "RT myRIO Target - Navigation\\Navi Global Variables.lvlib\\All Stop"(FALSE) -> ()  [unwired: 1 in, 1 out]
      n130 = call <vilib>:"Set Duty Cycle and Frequency.vi"("Frequency [Hz]"=w371, "Duty Cycle"=w370, "PWM Ref In"=w369) -> ("error out"=w376:errorcluster, "PWM Ref Out"=w383:T5)  [unwired: 6 in]
      n131 = call <vilib>:"Set Duty Cycle and Frequency.vi"("Frequency [Hz]"=w371, "Duty Cycle"=w370, "PWM Ref In"=w368) -> ("error out"=w381:errorcluster, "PWM Ref Out"=w382:T5)  [unwired: 6 in]
      n132 = call <vilib>:"Set Duty Cycle and Frequency.vi"("Frequency [Hz]"=w371, "Duty Cycle"=w370, "PWM Ref In"=w367) -> ("error out"=w375:errorcluster, "PWM Ref Out"=w380:T5)  [unwired: 6 in]
      n133 = call <vilib>:"Set Duty Cycle and Frequency.vi"("Frequency [Hz]"=w371, "Duty Cycle"=w370, "PWM Ref In"=w366) -> ("error out"=w374:errorcluster, "PWM Ref Out"=w379:T5)  [unwired: 6 in]
      n134 = call <vilib>:"Set Duty Cycle and Frequency.vi"("Frequency [Hz]"=w371, "Duty Cycle"=w370, "PWM Ref In"=w365) -> ("error out"=w373:errorcluster, "PWM Ref Out"=w378:T5)  [unwired: 6 in]
      n135 = call <vilib>:"Set Duty Cycle and Frequency.vi"("Frequency [Hz]"=w371, "Duty Cycle"=w370, "PWM Ref In"=w364) -> ("error out"=w372:errorcluster, "PWM Ref Out"=w377:T5)  [unwired: 6 in]
      n136 = local write "x position"(w361) -> ()
      n137 = local write "y position"(w361) -> ()
      n138 = call <vilib>:"Close.vi"("error in (no error)"=w376, "PWM Ref In"=w383) -> ()  [unwired: 9 in, 1 out]
      n139 = call <vilib>:"Close.vi"("error in (no error)"=w381, "PWM Ref In"=w382) -> ()  [unwired: 9 in, 1 out]
      n140 = call <vilib>:"Close.vi"("error in (no error)"=w375, "PWM Ref In"=w380) -> ()  [unwired: 9 in, 1 out]
      n141 = call <vilib>:"Close.vi"("error in (no error)"=w374, "PWM Ref In"=w379) -> ()  [unwired: 9 in, 1 out]
      n142 = call <vilib>:"Close.vi"("error in (no error)"=w373, "PWM Ref In"=w378) -> ()  [unwired: 9 in, 1 out]
      n143 = call <vilib>:"Close.vi"("error in (no error)"=w372, "PWM Ref In"=w377) -> ()  [unwired: 9 in, 1 out]
    }
  }
